vi "AlliGator Build Image SDV Profile Plots.vi"(0 "Intensity SDV":dbl[](array[numeric]), 1 "ROI Type":T4, 2 "Box Profile Type":T3, 3 "ROI Size String":string, 5 "Phase Lifetime SDV":dbl[](array[numeric]), 7 "Average Lifetime/Phasor Ratio SDV":dbl[](array[numeric]), 9 "Fit Parameter SDV":dbl[](array[numeric]), 11 "Error In":errorcluster, 12 "Fit Parameter Name":string, 13 "ratio(T)/<tau>(F)":bool, 14 "< t>_I (F)/<t>_A":bool) -> (4 "Plot Array":T1[](array[typedef]), 15 "Error Out":errorcluster)   [LabVIEW 2021, in "AlliGator Image Profile Window.lvlib"]
doc: "Builds the array of displayed SDV profiles according to the user-selected options and ROI type."
uses:
  AlliGator Image Profile Window.lvlib
  Image/Image ROI Type.ctl
  Image/Box Profile Type.ctl
  AlliGator Image Profile Plot Data.ctl
  Graphs/XY Graph/XY Plot Data.ctl
  Arrays/Linear Ramp End Options.ctl
  e9282ca8-7b4c-425d-bbd8-572d09d32eb6.vi
  52adedef-4fce-46da-a191-00be4efc5a4e.vi
  7c534c3e-da10-41db-a8ff-5ea6a11f1b7c.vi
  c62035f1-53a3-4edf-964a-62b160a8d83f.vi
  Graphs/XY Graph/XY Graph Add-Ons.lvlib
  Arrays/Arrays.lvlib
  Image/Image.lvlib
panel:
  # "see the AlliGator License on the block diagram (Ctrl+E or Window:Show Block Diagram)"
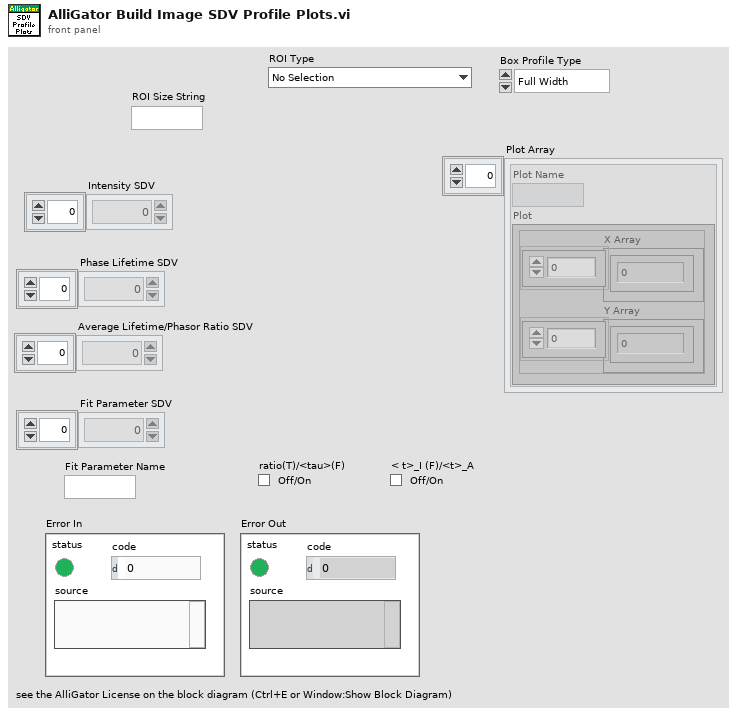
[diagram p1: front panel]
types:
  T1 = typedef "AlliGator Image Profile Window.lvlib/AlliGator Image Profile Plot Data.ctl" = cluster{"Plot Name":string, "Plot":T2}
  T2 = typedef "XY Graph Add-Ons.lvlib/XY Plot Data.ctl" = cluster{"X Array":dbl[], "Y Array":dbl[]}
  T3 = typedef "Image.lvlib/Box Profile Type.ctl" = enum16{"Full Width", "Half Width"}
  T4 = typedef "Image.lvlib/Image ROI Type.ctl" = enum16{"No Selection", "Point", "Line", "Rectangle", "Oval", "Polygon", "Freehand Region", "Annulus", "Unused2", "Unused3", "Broken Line", "Freehand Line", "Rotated Rectangle"}
  T5 = typedef "Arrays.lvlib/Linear Ramp End Options.ctl" = enum16{"Include Min/Exclude Max", "Exclude Min/Include Max", "Include Both Ends", "Exclude Both Ends"}
  T6 = cluster{"Ramp":dbl[], "Average Lifetime/Phasor Ratio SDV":dbl[]}
  T7 = cluster{"Ramp":dbl[], "Phase Lifetime SDV":dbl[]}
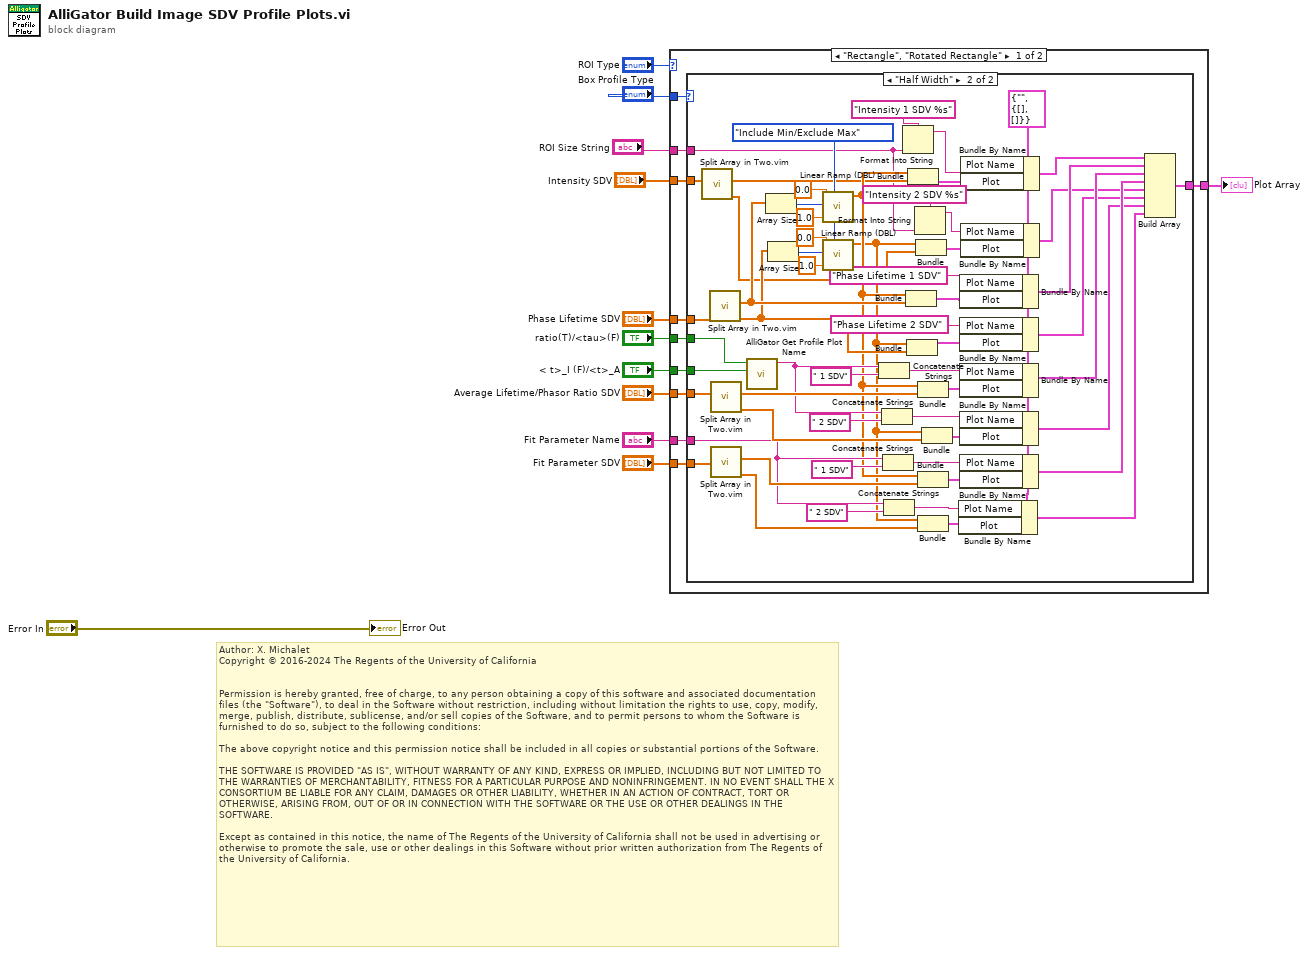
[diagram p0: block diagram]
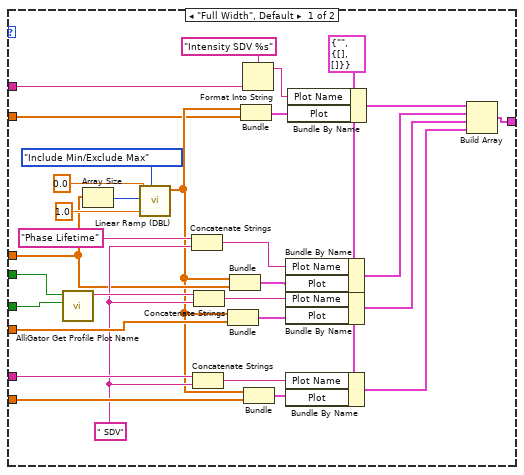
[diagram p2: hidden frame]
diagram:
  # "Author: X. Michalet\nCopyright © 2016-2024 The Regents of the University of California\n \n\nPermission is hereby granted, free of charge, to any person obtaining a copy of this software and associated documentation files (the \"Software\"), to deal in the Software without restriction, including without limitation the rights to use, copy, modify, merge, publish, distribute, sublicense, and/or sell copies of the Software, and to permit persons to whom the Software is furnished to do so, subject to the following conditions:\n\nThe above copyright notice and this permission notice shall be included in all copies or substantial portions of the Software.\n\nTHE SOFTWARE IS PROVIDED \"AS IS\", WITHOUT WARRANTY OF ANY KIND, EXPRESS OR IMPLIED, INCLUDING BUT NOT LIMITED TO THE WARRANTIES OF MERCHANTABILITY, FITNESS FOR A PARTICULAR PURPOSE AND NONINFRINGEMENT. IN NO EVENT SHALL THE X CONSORTIUM BE LIABLE FOR ANY CLAIM, DAMAGES OR OTHER LIABILITY, WHETHER IN AN ACTION OF CONTRACT, TORT OR OTHERWISE, ARISING FROM, OUT OF OR IN CONNECTION WITH THE SOFTWARE OR THE USE OR OTHER DEALINGS IN THE SOFTWARE.\n\nExcept as contained in this notice, the name of The Regents of the University of California shall not be used in advertising or otherwise to promote the sale, use or other dealings in this Software without prior written authorization from The Regents of the University of California."
  n1 = case shown="\"Rectangle\", \"Rotated Rectangle\"" "ROI Type" {
    tunnel: [w22 _] -> w4
    tunnel: "Average Lifetime/Phasor Ratio SDV" -> [w21 _]
    tunnel: "Fit Parameter SDV" -> [w20 _]
    tunnel: "Fit Parameter Name" -> [w19 _]
    tunnel: "< t>_I (F)/<t>_A" -> [w18 _]
    tunnel: "ratio(T)/<tau>(F)" -> [w17 _]
    tunnel: "Phase Lifetime SDV" -> [w16 _]
    tunnel: "Box Profile Type" -> [w15 _]
    tunnel: "Intensity SDV" -> [w14 _]
    tunnel: "ROI Size String" -> [w13 _]
    frame "Rectangle", "Rotated Rectangle" {
      n2 = case shown="\"Half Width\"" w15 {
        tunnel: [w49 w108] -> w22
        tunnel: w21 -> [w45 w90]
        tunnel: w20 -> [w42 w77]
        tunnel: w19 -> [w39 w74]
        tunnel: w18 -> [w37 w100]
        tunnel: w17 -> [w36 w99]
        tunnel: w16 -> [w31 w93]
        tunnel: w14 -> [w25 w60]
        tunnel: w13 -> [w24 w58]
        frame "Full Width", Default {
          w32 = " SDV" ("string")
          w28 = T1 {"Plot Name"="", "Plot"={"X Array"=[], "Y Array"=[]}} ("Plot Data")
          n3 = call "AlliGator Get Profile Plot Name.vi"("I-weighted (F)/A=weighted"=w37, "ratio(T)/<tau>(F)"=w36) -> ("Plot Name Suffix"=w38:string)  [unwired: 9 in]
          n4 = Array Size(array=w31) -> (size(s)=w50:i32)
          n5 = call "Linear Ramp (DBL).vi"("Options"=Linear_Ramp_End_Options."Include Min/Exclude Max", "Delta"=1.0, "Max"=w50, "Min"=0.0) -> ("Ramp"=w26:dbl[])  [unwired: 6 in, 1 out]
          n6 = Concatenate Strings("Phase Lifetime" ("Plot Name"), w32) -> (w35:string)
          n7 = Concatenate Strings(w39, w32) -> (w33:string)
          n8 = Concatenate Strings(w38, w32) -> (w34:string)
          n9 = Bundle("Ramp"=w26, "Average Lifetime/Phasor Ratio SDV"=w45) -> (w44:T6)  [unwired: 1 in]
          n10 = Bundle("Ramp"=w26, "Phase Lifetime SDV"=w31) -> (w48:T7)  [unwired: 1 in]
          n11 = Bundle("Ramp"=w26, "Intensity SDV"=w25) -> (w30:cluster{"Ramp":dbl[], "Intensity SDV":dbl[]})  [unwired: 1 in]
          n12 = Format Into String(format string="Intensity SDV %s" ("Plot Name"), w24) -> (resulting string=w29:string)  [unwired: 2 in, 1 out]
          n13 = Bundle("Ramp"=w26, "Fit Parameter SDV"=w42) -> (w41:cluster{"Ramp":dbl[], "Fit Parameter SDV":dbl[]})  [unwired: 1 in]
          n14 = Bundle By Name(cluster=w28, "Plot Name"=w35, "Plot"=w48) -> (w46:T1)
          n15 = Bundle By Name(cluster=w28, "Plot Name"=w34, "Plot"=w44) -> (w43:T1)
          n16 = Bundle By Name(cluster=w28, "Plot Name"=w33, "Plot"=w41) -> (w40:T1)
          n17 = Bundle By Name(cluster=w28, "Plot Name"=w29, "Plot"=w30) -> (w27:T1)
          n18 = Build Array(w27, w46, w43, w40) -> (w49:T1[])
        }
        frame "Half Width" {
          w95 = Linear_Ramp_End_Options."Include Min/Exclude Max" ("Options")
          w64 = T1 {"Plot Name"="", "Plot"={"X Array"=[], "Y Array"=[]}} ("Plot Data")
          n19 = call "Split Array in Two.vim"("Array in"=w60) -> ("Second Half Array"=w56:dbl[], "First Half Array"=w59:dbl[])  [unwired: 9 in]
          n20 = call "Split Array in Two.vim"("Array in"=w93) -> ("Second Half Array"=w69:dbl[], "First Half Array"=w70:dbl[])  [unwired: 9 in]
          n21 = call "Split Array in Two.vim"("Array in"=w90) -> ("Second Half Array"=w87:dbl[], "First Half Array"=w89:dbl[])  [unwired: 9 in]
          n22 = call "Split Array in Two.vim"("Array in"=w77) -> ("Second Half Array"=w71:dbl[], "First Half Array"=w78:dbl[])  [unwired: 9 in]
          n23 = call "AlliGator Get Profile Plot Name.vi"("I-weighted (F)/A=weighted"=w100, "ratio(T)/<tau>(F)"=w99) -> ("Plot Name Suffix"=w83:string)  [unwired: 9 in]
          n24 = Array Size(array=w70) -> (size(s)=w109:i32)
          n25 = Array Size(array=w69) -> (size(s)=w98:i32)
          n26 = call "Linear Ramp (DBL).vi"("Options"=w95, "Delta"=1.0, "Max"=w109, "Min"=0.0) -> ("Ramp"=w61:dbl[])  [unwired: 6 in, 1 out]
          n27 = call "Linear Ramp (DBL).vi"("Options"=w95, "Delta"=1.0, "Max"=w98, "Min"=0.0) -> ("Ramp"=w57:dbl[])  [unwired: 6 in, 1 out]
          n28 = Concatenate Strings(w83, " 1 SDV" ("string")) -> (w86:string)
          n29 = Concatenate Strings(w83, " 2 SDV" ("string")) -> (w82:string)
          n30 = Concatenate Strings(w74, " 1 SDV" ("string")) -> (w79:string)
          n31 = Concatenate Strings(w74, " 2 SDV" ("string")) -> (w75:string)
          n32 = Format Into String(format string="Intensity 1 SDV %s" ("Plot Name"), w58) -> (resulting string=w66:string)  [unwired: 2 in, 1 out]
          n33 = Bundle("Ramp"=w61, "First Half Array"=w70) -> (w107:cluster{"Ramp":dbl[], "First Half Array":dbl[]})  [unwired: 1 in]
          n34 = Bundle("Ramp"=w57, "Second Half Array"=w69) -> (w92:cluster{"Ramp":dbl[], "Second Half Array":dbl[]})  [unwired: 1 in]
          n35 = Bundle("Ramp"=w61, "First Half Array"=w59) -> (w68:cluster{"Ramp":dbl[], "First Half Array":dbl[]})  [unwired: 1 in]
          n36 = Format Into String(format string="Intensity 2 SDV %s" ("Plot Name"), w58) -> (resulting string=w65:string)  [unwired: 2 in, 1 out]
          n37 = Bundle("Ramp"=w57, "Second Half Array"=w56) -> (w67:cluster{"Ramp":dbl[], "Second Half Array":dbl[]})  [unwired: 1 in]
          n38 = Bundle("Ramp"=w61, "First Half Array"=w89) -> (w104:cluster{"Ramp":dbl[], "First Half Array":dbl[]})  [unwired: 1 in]
          n39 = Bundle("Ramp"=w61, "First Half Array"=w78) -> (w102:cluster{"Ramp":dbl[], "First Half Array":dbl[]})  [unwired: 1 in]
          n40 = Bundle("Ramp"=w57, "Second Half Array"=w71) -> (w76:cluster{"Ramp":dbl[], "Second Half Array":dbl[]})  [unwired: 1 in]
          n41 = Bundle("Ramp"=w57, "Second Half Array"=w87) -> (w88:cluster{"Ramp":dbl[], "Second Half Array":dbl[]})  [unwired: 1 in]
          n42 = Bundle By Name(cluster=w64, "Plot Name"=w75, "Plot"=w76) -> (w72:T1)
          n43 = Bundle By Name(cluster=w64, "Plot Name"="Phase Lifetime 1 SDV", "Plot"=w107) -> (w105:T1)
          n44 = Bundle By Name(cluster=w64, "Plot Name"="Phase Lifetime 2 SDV", "Plot"=w92) -> (w91:T1)
          n45 = Bundle By Name(cluster=w64, "Plot Name"=w86, "Plot"=w104) -> (w103:T1)
          n46 = Bundle By Name(cluster=w64, "Plot Name"=w82, "Plot"=w88) -> (w81:T1)
          n47 = Bundle By Name(cluster=w64, "Plot Name"=w79, "Plot"=w102) -> (w101:T1)
          n48 = Bundle By Name(cluster=w64, "Plot Name"=w66, "Plot"=w68) -> (w63:T1)
          n49 = Bundle By Name(cluster=w64, "Plot Name"=w65, "Plot"=w67) -> (w55:T1)
          n50 = Build Array(w63, w105, w103, w101, w55, w91, w81, w72) -> (w108:T1[])
        }
      }
    }
    frame "Oval", Default {
    }
  }
  "Plot Array" <- w4
  "Error Out" <- "Error In"
